vi "Vspeed adjust (SubVI).vi"(11 "Y":sgl) -> (1 "Boolean":bool, 2 "Numeric":dbl, 3 "Boolean 2":bool)   [LabVIEW 2014]
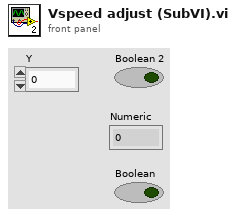
[diagram p1: front panel]
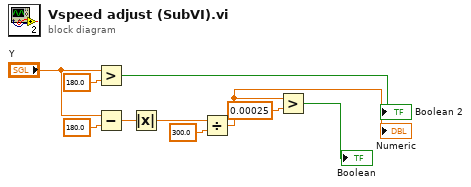
[diagram p0: block diagram]
diagram:
  n1 = Greater?(x="Y", y=180.0) -> (0:→"Boolean 2":bool)
  n2 = Subtract(x="Y", y=180.0) -> (x-y=w4:dbl)
  n3 = Absolute Value(x=w4) -> (abs(x)=w5:dbl)
  n4 = Divide(x=w5, y=300.0) -> (x/y=w8:dbl)
  "Numeric" <- w8
  n5 = Greater?(x=w8, y=0.00025) -> (0:→"Boolean":bool)
